vi "Set Configuration File.vi"(8 "error in (no error)":errorcluster) -> (0 "error out":errorcluster, 1 "DIAdem?":bool)   [LabVIEW 2011]
uses:
  ITK EXT/utils/strutil.llb/Case Matching.ctl
  Spartan CONFIG Global.vi
  Spartan Version.vi
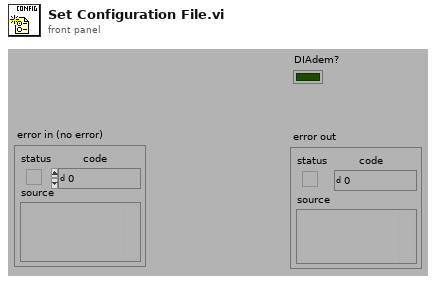
[diagram p1: front panel]
types:
  T1 = typedef "Case Matching.ctl" = enum16{"a != A", "a == A", "system"}
  T2 = enum32{"invalid app kind", "Development System", "Run Time System", "Student Edition", "Embedded LabVIEW", "Evaluation", "Custom"}
  T3 = typedef "Keyed Array.ctl" = cluster{"keys":string[], "values":string[]}
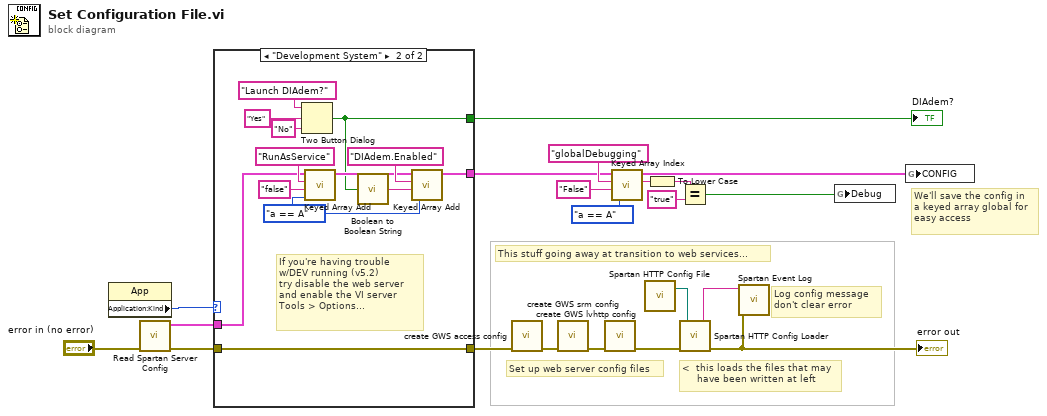
[diagram p0: block diagram]
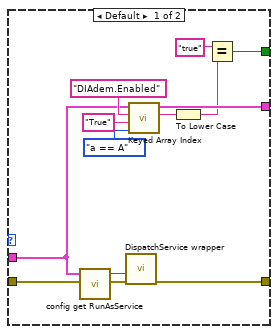
[diagram p2: hidden frame]
diagram:
  # "Log config message\ndon't clear error"
  # "<  this loads the files that may\n     have been written at left"
  # "Set up web server config files"
  # "This stuff going away at transition to web services..."
  # "We'll save the config in\na keyed array global for\neasy access"
  n1 = property class="App"() -> ("Application:Kind"=w15:T2)  [unwired: 2 in, 2 out]
  n2 = call "Read Spartan Server Config.vi"("error in (no error)"="error in (no error)") -> ("error out"=w3:errorcluster, "Config Keys"=w5:T3)  [unwired: 5 in]
  n3 = case shown="\"Development System\"" w15 {
    tunnel: w5 -> [w25 w41]
    tunnel: [w26 w38] -> w14
    tunnel: w3 -> [w33 w35]
    tunnel: [w32 w35] -> w2
    tunnel: [w24 w36] -> w1
    frame Default {
      n4 = call "config get RunAsService.vi"("Config Keys"=w25) -> ("RunAsService?"=w31:bool)  [unwired: 4 out]
      n5 = call "DispatchService wrapper.vi"("error in (no error)"=w33, "Dispatch Service? (f)"=w31) -> ("error out"=w32:errorcluster)  [unwired: 9 out]
      n6 = call "Keyed Array Index.vi"("case matching (sensitive)"=Case_Matching."a == A", "default value"="True", "key"="DIAdem.Enabled", "array in"=w25) -> ("value"=w27:string, "duplicate array"=w26:T3)  [unwired: 2 out]
      n7 = To Lower Case(string=w27) -> (all lower case string=w23:string)
      n8 = Equal?(x="true" ("y"), y=w23) -> (x = y?=w24:bool)
    }
    frame "Development System" {
      w34 = Case_Matching."a == A" ("case matching (sensitive)")
      # "If you're having trouble\nw/DEV running (v5.2)\ntry disable the web server\nand enable the VI server\nTools > Options..."
      n9 = Two Button Dialog(message="Launch DIAdem?", 1:"No", 2:"Yes") -> (T button?=w36:bool)
      n10 = call "Keyed Array Add.vi"("case matching (sensitive)"=w34, "value"="false", "key"="RunAsService" ("value"), "array in"=w41) -> ("array out"=w39:T3)  [unwired: 3 out]
      n11 = call "Boolean to Boolean String.vi"("Boolean"=w36) -> ("Boolean string"=w37:string)  [unwired: 1 in]
      n12 = call "Keyed Array Add.vi"("case matching (sensitive)"=w34, "value"=w37, "key"="DIAdem.Enabled" ("value"), "array in"=w39) -> ("array out"=w38:T3)  [unwired: 3 out]
    }
  }
  "DIAdem?" <- w1
  n13 = call "create GWS access config.vi"("error in (no error)"=w2) -> ("error out"=w12:errorcluster)  [unwired: 6 out]
  n14 = call "create GWS srm config.vi"("error in (no error)"=w12) -> ("error out"=w11:errorcluster)  [unwired: 6 out]
  n15 = call "create GWS lvhttp config.vi"("error in (no error)"=w11) -> ("error out"=w9:errorcluster)  [unwired: 6 out]
  n16 = call "Keyed Array Index.vi"("case matching (sensitive)"=Case_Matching."a == A", "default value"="False", "key"="globalDebugging", "array in"=w14) -> ("value"=w18:string, "duplicate array"=w4:T3)  [unwired: 2 out]
  n17 = call "Spartan HTTP Config File.vi"() -> ("HTTP Configuration File"=w10:path)  [unwired: 1 out]
  n18 = To Lower Case(string=w18) -> (all lower case string=w16:string)
  n19 = Equal?(x=w16, y="true") -> (x = y?=w13:bool)
  n20 = call "Spartan HTTP Config Loader.vi"("error in (no error)"=w9, "lvhttp.cfg"=w10) -> ("error out"=w7:errorcluster, "Config Load Message"=w8:string)  [unwired: 4 out]
  "error out" <- w7
  n21 = call "Spartan Event Log.vi"("error in (no error)"=w7, "message (\"\")"=w8) -> ()  [unwired: 3 in, 4 out]
  n22 = global write "Spartan Version.vi" "Debug"(w13) -> ()
  n23 = global write "Spartan CONFIG Global.vi" "CONFIG"(w4) -> ()
